vi "Get RT Data.vi"(8 "error in (no error)":errorcluster, 11 "RT SubAddresses XML Ref":refnum<k20>[](array[refnum])) -> (0 "error out":errorcluster, 3 "SubAddress Configurations":T1[](array[typedef]) {"Data Fields"."Base Word" format="%04x"; "Data Fields"."Address" format="%016x"; "Data Fields"."Mask" format="%04x"; "Data Fields"."Value" format="%016x"; "Data" format="%04x"})   [LabVIEW 2016]
doc: "Retrieves all the settings for the subaddresses defined for a single Remote Terminal on a Component."
uses:
  <vilib>/xml/NI_XML.lvlib
  1553 SubComponent/TypeDefs/Scaling Information.ctl
  1553 SubComponent/1553 SubComponent.lvclass
  1553 SubComponent/TypeDefs/Parameter Table Data.ctl
  Remote Terminal/TypeDefs/Command Type.ctl
  Remote Terminal/Remote Terminal.lvclass
  Remote Terminal/TypeDefs/Command Configuration.ctl
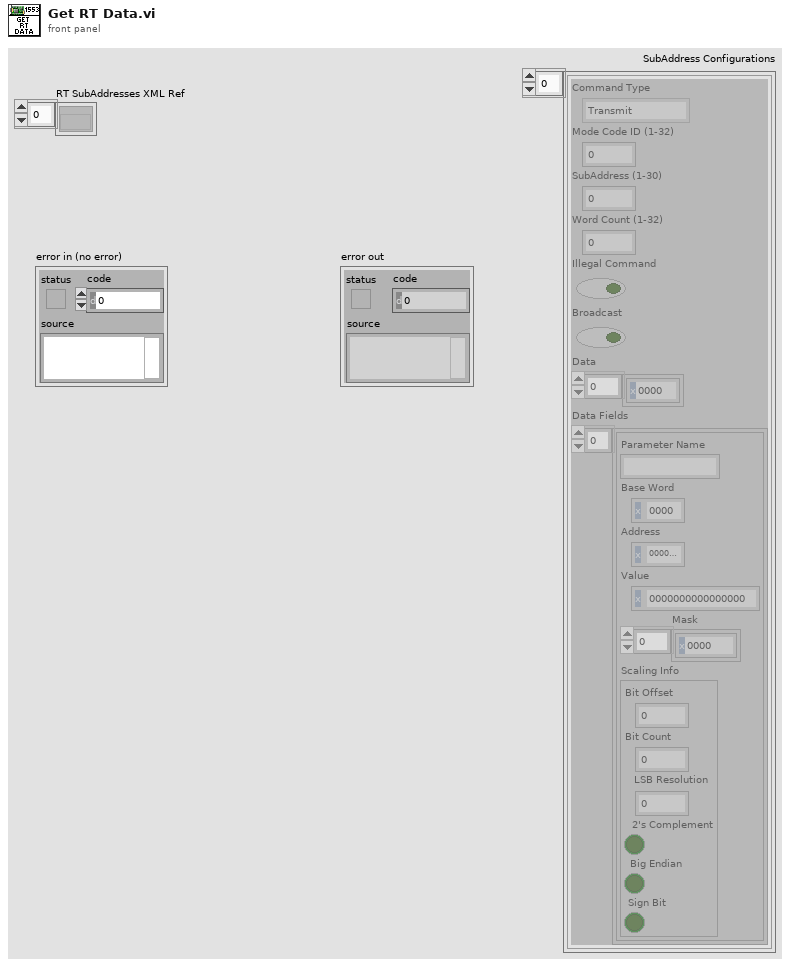
[diagram p1: front panel]
types:
  T1 = typedef "BCI-1553 API.lvlib/Remote Terminal.lvclass/Command Configuration.ctl" = cluster{"Command Type":T2, "Mode Code ID (1-32)":u16, "SubAddress (1-30)":u16, "Word Count (1-32)":u16, "Illegal Command":bool, "Broadcast":bool, "Data":u16[], "Data Fields":T3[]}
  T2 = typedef "BCI-1553 API.lvlib/Remote Terminal.lvclass/Command Type.ctl" = enum16{"Transmit", "Receive", "Mode Code Tx", "Mode Code Rx"}
  T3 = typedef "BCI-1553 API.lvlib/1553 SubComponent.lvclass/Parameter Table Data.ctl" = cluster{"Parameter Name":string, "Base Word":u16, "Address":u16, "Value":u64, "Mask":u16[], "Scaling Info":T4}
  T4 = typedef "BCI-1553 API.lvlib/1553 SubComponent.lvclass/Scaling Information.ctl" = cluster{"Bit Offset":i32, "Bit Count":i32, "LSB Resolution":dbl, "2's Complement":bool, "Big Endian":bool, "Sign Bit":bool}
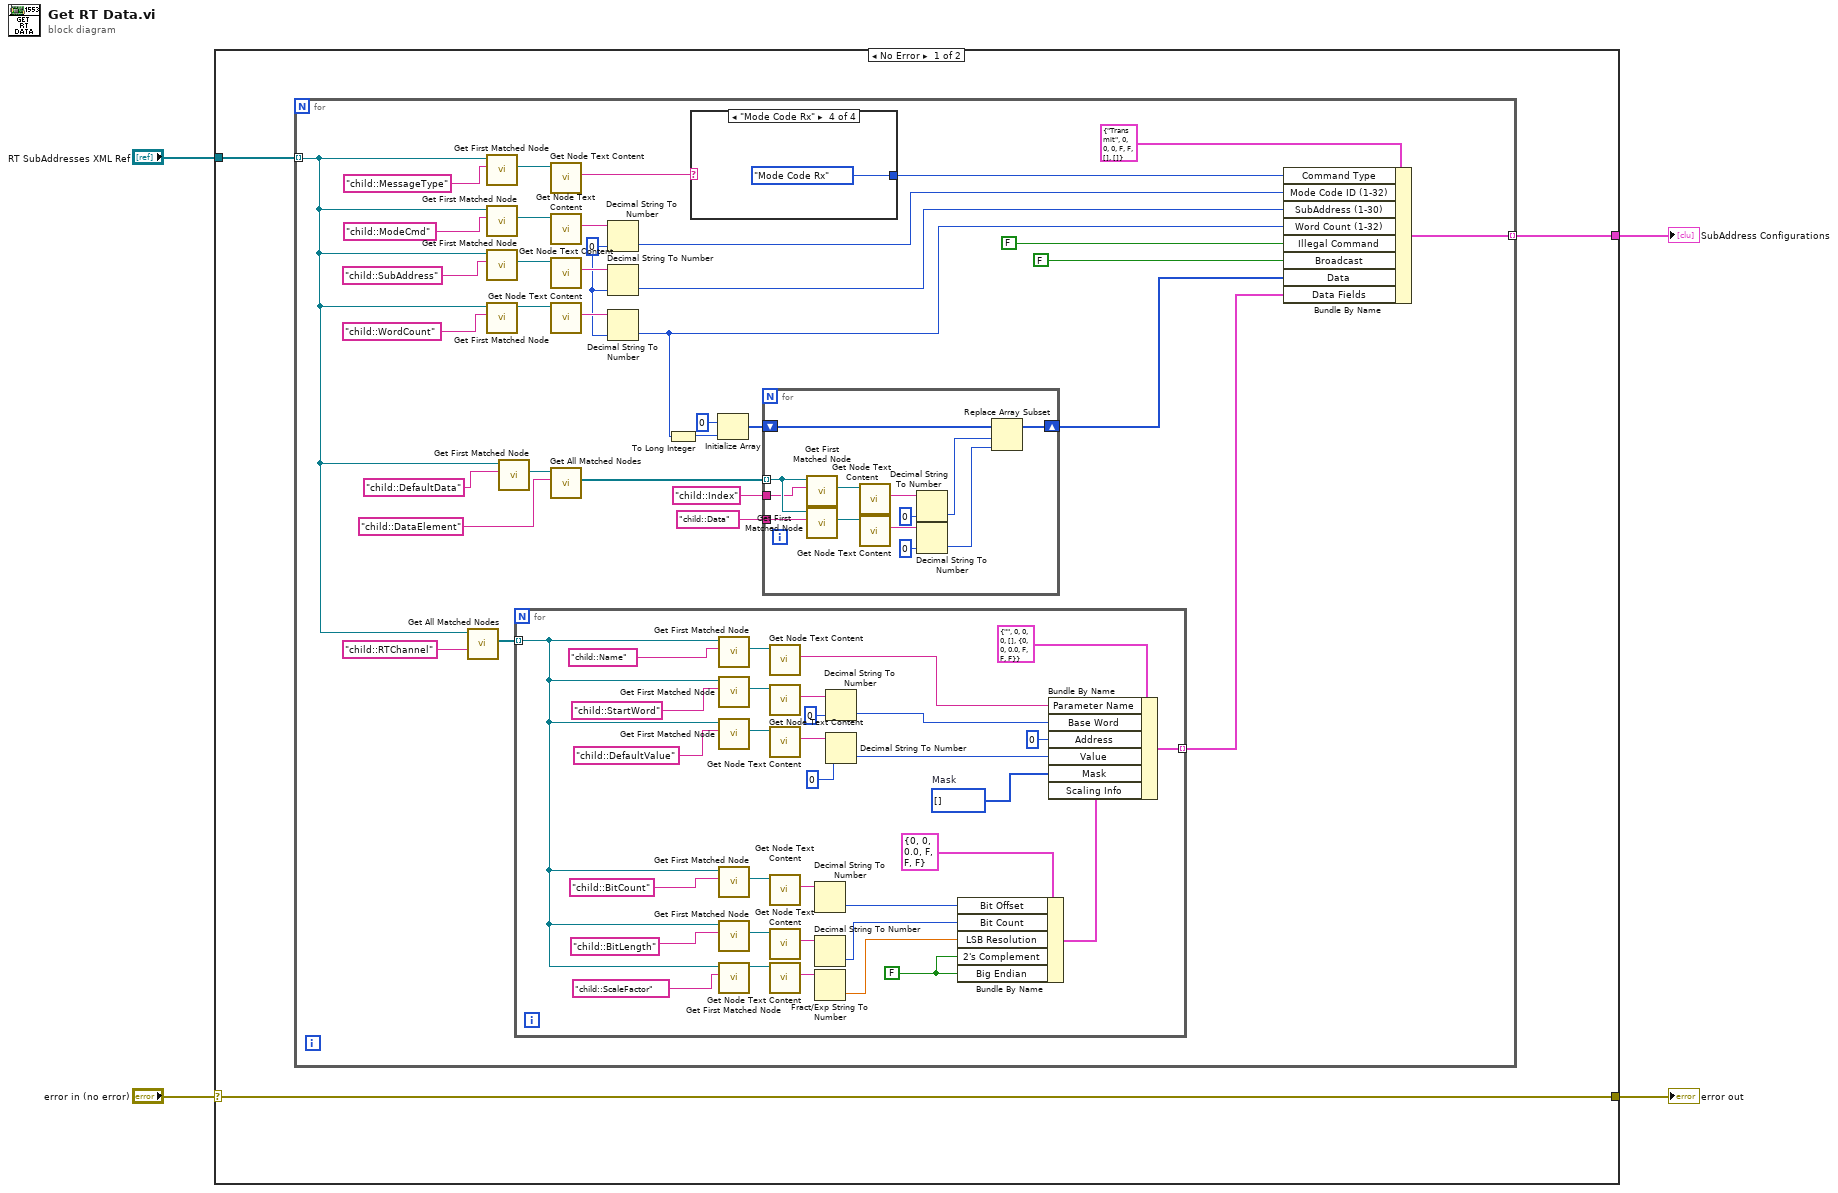
[diagram p0: block diagram]
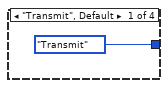
[diagram p2: hidden frame]
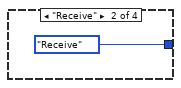
[diagram p3: hidden frame]
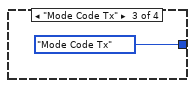
[diagram p4: hidden frame]
diagram:
  n1 = case shown="No Error" "error in (no error)" {
    selector: "error in (no error)" -> [w5 w93]
    tunnel: "RT SubAddresses XML Ref" -> [w7 _]
    tunnel: [w6 _] -> w3
    tunnel: [w5 w93] -> w1
    frame No Error {
      n2 = for {
        tunnel: w7 -> [w9] mode=indexing
        tunnel: [w20] -> w6 mode=indexing
        w25 = u16 0 ("default (0 I32)")
        n3 = call <vilib>:"Get All Matched Nodes.vi"("XPath expression"="child::RTChannel", "node in"=w9) -> ("node result array"=w29:refnum<k20>[])  [unwired: 7 in, 2 out]
        n4 = call <vilib>:"Get First Matched Node.vi"("XPath expression"="child::MessageType", "node in"=w9) -> ("node result"=w37:refnum<k20>)  [unwired: 7 in, 2 out]
        n5 = call <vilib>:"Get First Matched Node.vi"("XPath expression"="child::ModeCmd", "node in"=w9) -> ("node result"=w35:refnum<k20>)  [unwired: 7 in, 2 out]
        n6 = call <vilib>:"Get First Matched Node.vi"("XPath expression"="child::SubAddress", "node in"=w9) -> ("node result"=w32:refnum<k20>)  [unwired: 7 in, 2 out]
        n7 = call <vilib>:"Get First Matched Node.vi"("XPath expression"="child::WordCount", "node in"=w9) -> ("node out"=w31:refnum<k20>)  [unwired: 7 in, 2 out]
        n8 = call <vilib>:"Get First Matched Node.vi"("XPath expression"="child::DefaultData", "node in"=w9) -> ("node result"=w13:refnum<k20>)  [unwired: 7 in, 2 out]
        n9 = for {
          tunnel: w29 -> [w77] mode=indexing
          tunnel: [w60] -> w21 mode=indexing
          w67 = u16[] []  # Mask
          w70 = FALSE
          n10 = call <vilib>:"Get First Matched Node.vi"("XPath expression"="child::Name", "node in"=w77) -> ("node result"=w80:refnum<k20>)  [unwired: 7 in, 2 out]
          n11 = call <vilib>:"Get First Matched Node.vi"("XPath expression"="child::StartWord", "node in"=w77) -> ("node result"=w79:refnum<k20>)  [unwired: 7 in, 2 out]
          n12 = call <vilib>:"Get First Matched Node.vi"("XPath expression"="child::DefaultValue", "node in"=w77) -> ("node result"=w82:refnum<k20>)  [unwired: 7 in, 2 out]
          n13 = call <vilib>:"Get First Matched Node.vi"("XPath expression"="child::BitCount", "node in"=w77) -> ("node result"=w89:refnum<k20>)  [unwired: 7 in, 2 out]
          n14 = call <vilib>:"Get First Matched Node.vi"("XPath expression"="child::BitLength", "node in"=w77) -> ("node result"=w90:refnum<k20>)  [unwired: 7 in, 2 out]
          n15 = call <vilib>:"Get First Matched Node.vi"("XPath expression"="child::ScaleFactor", "node in"=w77) -> ("node out"=w86:refnum<k20>)  [unwired: 7 in, 2 out]
          n16 = call <vilib>:"Get Node Text Content.vi"("node in"=w80) -> ("node text"=w62:string)  [unwired: 8 in, 2 out]
          n17 = call <vilib>:"Get Node Text Content.vi"("node in"=w79) -> ("node text"=w75:string)  [unwired: 8 in, 2 out]
          n18 = call <vilib>:"Get Node Text Content.vi"("node in"=w82) -> ("node text"=w76:string)  [unwired: 8 in, 2 out]
          n19 = call <vilib>:"Get Node Text Content.vi"("node in"=w89) -> ("node text"=w91:string)  [unwired: 8 in, 2 out]
          n20 = call <vilib>:"Get Node Text Content.vi"("node in"=w90) -> ("node text"=w92:string)  [unwired: 8 in, 2 out]
          n21 = call <vilib>:"Get Node Text Content.vi"("node in"=w86) -> ("node text"=w84:string)  [unwired: 8 in, 2 out]
          n22 = Decimal String To Number(string=w91) -> (number=w73:i32)  [unwired: 2 in, 1 out]
          n23 = Decimal String To Number(string=w92) -> (number=w72:i32)  [unwired: 2 in, 1 out]
          n24 = Fract/Exp String To Number(string=w84) -> (number=w71:dbl)  [unwired: 3 in, 1 out]
          n25 = Decimal String To Number(string=w75, default (0L)=u16 0 ("default (0 I32)")) -> (number=w64:u16)  [unwired: 1 in, 1 out]
          n26 = Decimal String To Number(string=w76, default (0L)=u64 0 ("default (0 I32)")) -> (number=w65:u64)  [unwired: 1 in, 1 out]
          n27 = Bundle By Name(cluster=T4 {"Bit Offset"=0, "Bit Count"=0, "LSB Resolution"=0.0, "2's Complement"=FALSE, "Big Endian"=FALSE, "Sign Bit"=FALSE} ("Scaling Info"), "Bit Offset"=w73, "Bit Count"=w72, "LSB Resolution"=w71, "2's Complement"=w70, "Big Endian"=w70) -> (w68:T4)
          n28 = Bundle By Name(cluster=T3 {"Parameter Name"="", "Base Word"=0, "Address"=0, "Value"=0, "Mask"=[], "Scaling Info"={"Bit Offset"=0, "Bit Count"=0, "LSB Resolution"=0.0, "2's Complement"=FALSE, "Big Endian"=FALSE, "Sign Bit"=FALSE}} ("Parameter Table Data"), "Parameter Name"=w62, "Base Word"=w64, "Address"=u16 0, "Value"=w65, "Mask"=w67, "Scaling Info"=w68) -> (w60:T3)
        }
        n29 = call <vilib>:"Get Node Text Content.vi"("node in"=w37) -> ("node text"=w36:string)  [unwired: 8 in, 2 out]
        n30 = call <vilib>:"Get Node Text Content.vi"("node in"=w35) -> ("node text"=w34:string)  [unwired: 8 in, 2 out]
        n31 = call <vilib>:"Get Node Text Content.vi"("node in"=w32) -> ("node text"=w33:string)  [unwired: 8 in, 2 out]
        n32 = call <vilib>:"Get Node Text Content.vi"("node in"=w31) -> ("node text"=w30:string)  [unwired: 8 in, 2 out]
        n33 = call <vilib>:"Get All Matched Nodes.vi"("XPath expression"="child::DataElement", "node in"=w13) -> ("node result array"=w11:refnum<k20>[])  [unwired: 7 in, 2 out]
        n34 = Decimal String To Number(string=w34, default (0L)=w25) -> (number=w26:u16)  [unwired: 1 in, 1 out]
        n35 = Decimal String To Number(string=w33, default (0L)=w25) -> (number=w24:u16)  [unwired: 1 in, 1 out]
        n36 = Decimal String To Number(string=w30, default (0L)=w25) -> (number=w10:u16)  [unwired: 1 in, 1 out]
        n37 = To Long Integer(number=w10) -> (32bit integer=w16:i32)
        n38 = case shown="\"Mode Code Rx\"" w36 {
          tunnel: [Command_Type."Transmit" ("Command Type") Command_Type."Receive" ("Command Type") Command_Type."Mode Code Tx" ("Command Type") Command_Type."Mode Code Rx" ("Command Type")] -> w27
          frame "Transmit", Default {
          }
          frame "Receive" {
          }
          frame "Mode Code Tx" {
          }
          frame "Mode Code Rx" {
          }
        }
        n39 = Initialize Array(u16 0 ("element"), w16) -> (w15:u16[])
        n40 = for {
          tunnel: w11 -> [w53] mode=indexing
          shift-right: [w54] -> w8
          shift-left: w15 -> [w55]
          tunnel: "child::Index" ("XPath expression") -> [w52]
          tunnel: "child::Data" ("XPath expression") -> [w51]
          n41 = call <vilib>:"Get First Matched Node.vi"("XPath expression"=w52, "node in"=w53) -> ("node result"=w50:refnum<k20>)  [unwired: 7 in, 2 out]
          n42 = call <vilib>:"Get First Matched Node.vi"("XPath expression"=w51, "node in"=w53) -> ("node result"=w49:refnum<k20>)  [unwired: 7 in, 2 out]
          n43 = call <vilib>:"Get Node Text Content.vi"("node in"=w50) -> ("node text"=w46:string)  [unwired: 8 in, 2 out]
          n44 = call <vilib>:"Get Node Text Content.vi"("node in"=w49) -> ("node text"=w45:string)  [unwired: 8 in, 2 out]
          n45 = Decimal String To Number(string=w46, default (0L)=0 ("Command Config.Terminal Address (0-30)")) -> (number=w44:i32)  [unwired: 1 in, 1 out]
          n46 = Decimal String To Number(string=w45, default (0L)=u16 0 ("Command Config.Terminal Address (0-30)")) -> (number=w43:u16)  [unwired: 1 in, 1 out]
          n47 = Replace Array Subset(array=w55, new element=w43, index=w44) -> (w54:u16[])
        }
        n48 = Bundle By Name(cluster=T1 {"Command Type"=enum."Transmit", "Mode Code ID (1-32)"=0, "SubAddress (1-30)"=0, "Word Count (1-32)"=0, "Illegal Command"=FALSE, "Broadcast"=FALSE, "Data"=[], "Data Fields"=[]} ("CMD Configuration"), "Command Type"=w27, "Mode Code ID (1-32)"=w26, "SubAddress (1-30)"=w24, "Word Count (1-32)"=w10, "Illegal Command"=FALSE, "Broadcast"=FALSE, "Data"=w8, "Data Fields"=w21) -> (w20:T1)
      }
    }
    frame Error {
    }
  }
  "error out" <- w1
  "SubAddress Configurations" <- w3
